vi "sub04_ReadPos.vi"() -> ()   [LabVIEW 2019]
panel:
  out "cancelled":bool
  out "error out":errorcluster
  out "text":string
  out "refnum out":refnum<file>
  in  "error in":errorcluster
  in  "file (use dialog)":path
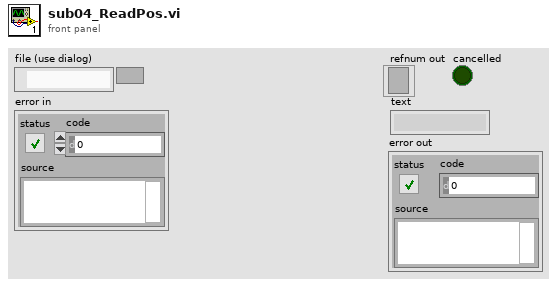
[diagram p1: front panel]
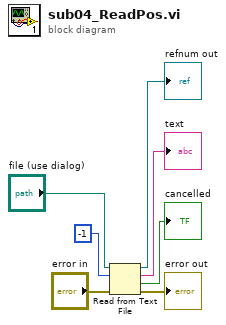
[diagram p0: block diagram]
diagram:
  n1 = Read from Text File(file (use dialog)="file (use dialog)", count=-1, error in="error in") -> (refnum out=→"refnum out":refnum<file>, text=→"text":string, cancelled=→"cancelled":bool, error out=→"error out":errorcluster)  [unwired: 1 in]
